vi "Write DAQ Data.vi"(8 "error in (no error)":errorcluster, 9 "Voltage with Time":dbl[][](array[numeric]), 10 "File Infor":T1, 11 "File Manager in":refnum<class "File Abstract.lvclass">) -> (0 "error out":errorcluster, 3 "File Manager out":refnum<class "File Abstract.lvclass">)   [LabVIEW 2021, in "File Abstract.lvclass"]
doc: "Do nothing."
uses:
  File Abstract.lvclass
  Control/File Information Cluster.ctl
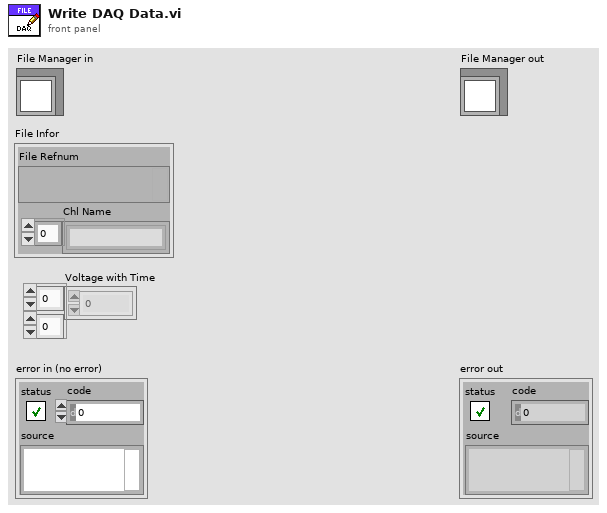
[diagram p1: front panel]
types:
  T1 = typedef "File Information Cluster.ctl" = cluster{"File Refnum":variant, "Chl Name":string[]}
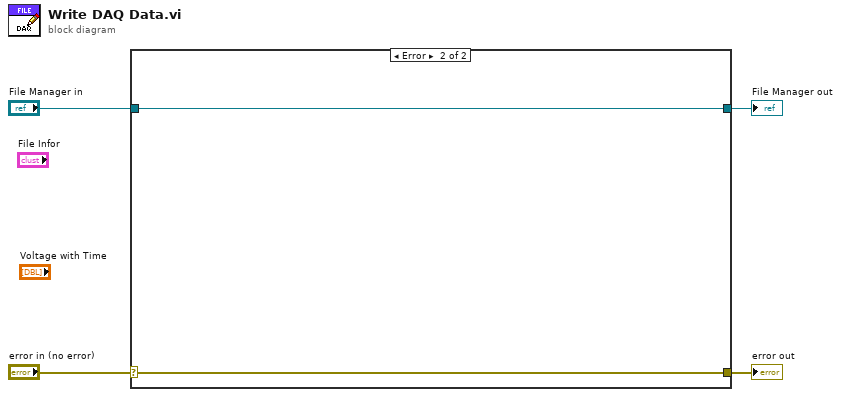
[diagram p0: block diagram]
diagram:
  n1 = case shown="Error" "error in (no error)" {
    selector: "error in (no error)" -> [w6 w8]
    tunnel: [w6 w8] -> w3
    tunnel: [w5 w7] -> w1
    tunnel: "File Manager in" -> [w5 w7]
    frame No Error {
      # "Wire the error cluster across even in the \"No Error\"\ncase so that warnings get propagated."
    }
    frame Error {
    }
  }
  "error out" <- w3
  "File Manager out" <- w1
